vi "Test Client.vi"() -> ()   [LabVIEW 2018, in "InfluxDB Client.lvlib"]
doc: "Test program for the InfluxDB client."
uses:
  Controls/FieldSet.ctl
  Controls/TagSet.ctl
  Controls/Precision.ctl
  Classes/DataPoint/DataPoint.lvclass/DataPoint.ctl
  Classes/Results/Results.lvclass/Results.ctl
  Classes/Result/Result.lvclass/Result.ctl
  Classes/Series/Series.lvclass/Series.ctl
  InfluxDB Client.lvlib
  Classes/Client/Client.lvclass
  Classes/DataPoint/DataPoint.lvclass
  Classes/Results/Results.lvclass
  Classes/Result/Result.lvclass
  Classes/Series/Series.lvclass
panel:
  out "Tag keys":string[][][](array[string])
  out "Field keys":string[][][](array[string])
  out "Version":string
  out "Values":string[][](array[string])
  out "error out":errorcluster
  out "Measurement names":string[](array[string])
  out "Database names":string[](array[string])
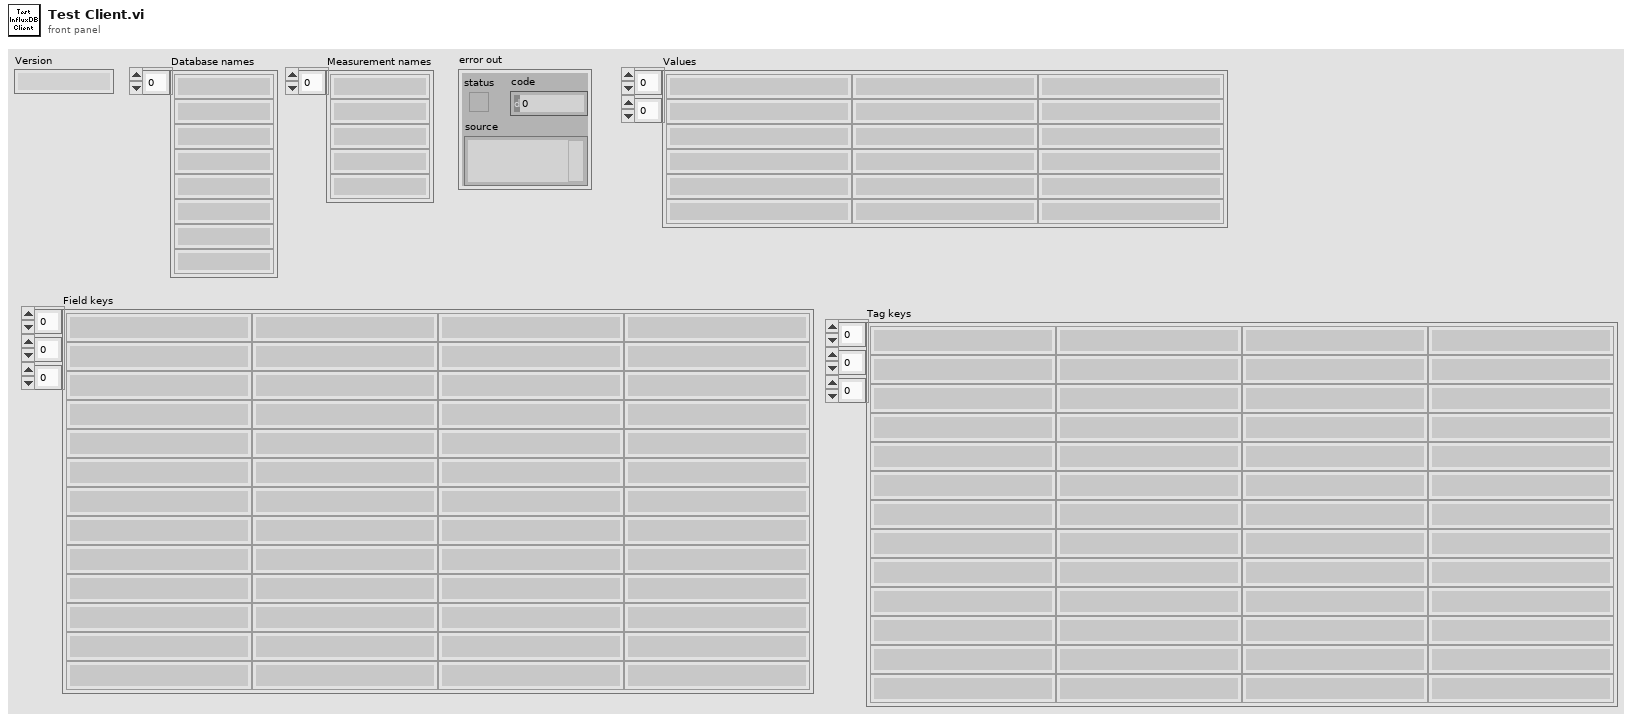
[diagram p1: front panel]
types:
  T1 = typedef "InfluxDB Client.lvlib/Precision.ctl" = enum16{"Seconds", "Milliseconds", "Nanoseconds"}
  T2 = typedef "InfluxDB Client.lvlib/TagSet.ctl" = cluster{"Key":string, "Value":string}
  T3 = typedef "InfluxDB Client.lvlib/FieldSet.ctl" = cluster{"Key":string, "Value":variant}
  T4 = typedef "Dictionary Object RefNum__ogtk.ctl" = refnum<k1>
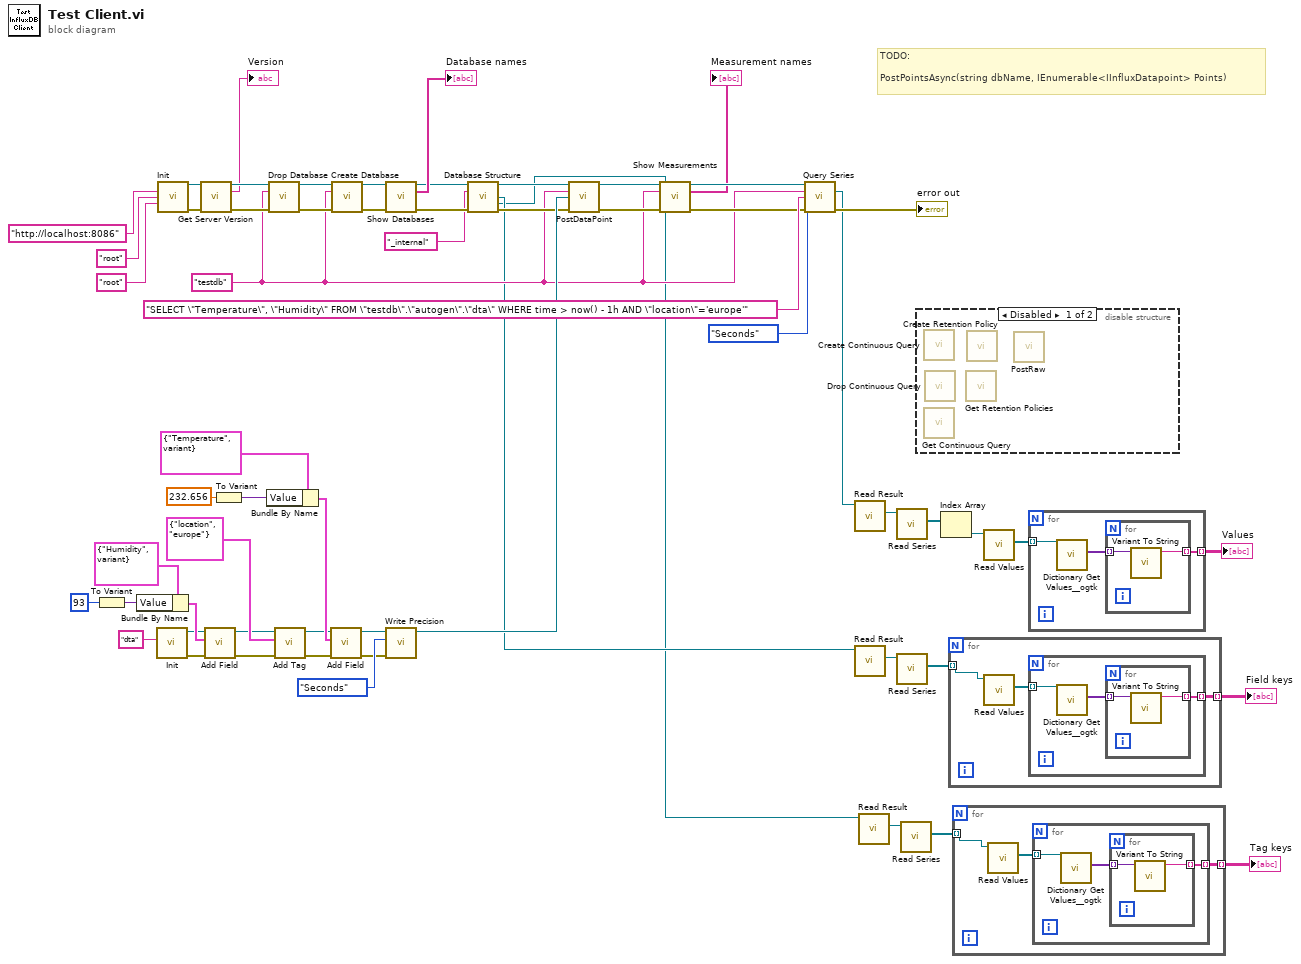
[diagram p0: block diagram]
diagram:
  w10 = "testdb" ("Database name")
  # "TODO:\n\nPostPointsAsync(string dbName, IEnumerable<IInfluxDatapoint> Points)"
  n1 = To Variant(anything=i8 93) -> (Variant=w52:variant)
  n2 = Bundle By Name(cluster=T3 {"Key"="Humidity", "Value"=variant} ("FieldSet"), "Value"=w52) -> (w51:T3)
  n3 = call "Init.vi"("Measurement"="dta") -> ("error out"=w44:errorcluster, "DataPoint out"=w45:refnum<class "DataPoint.lvclass">)  [unwired: 9 in]
  n4 = call "Init.vi"("Url"="http://localhost:8086", "Username"="root" ("Url"), "Password"="root" ("Url")) -> ("InfluxDB out"=w39:refnum<class "Client.lvclass">, "error out"=w38:errorcluster)  [unwired: 11 in]
  n5 = call "Get Server Version.vi"("InfluxDB in"=w39, "error in (no error)"=w38) -> ("InfluxDB out"=w27:refnum<class "Client.lvclass">, "Version"=→"Version":string, "error out"=w26:errorcluster)  [unwired: 11 in]
  n6 = call "Add Field.vi"("error in (no error)"=w44, "FieldSet"=w51, "DataPoint in"=w45) -> ("error out"=w42:errorcluster, "DataPoint out"=w43:refnum<class "DataPoint.lvclass">)  [unwired: 7 in]
  n7 = To Variant(anything=232.656 ("temperature")) -> (Variant=w50:variant)
  n8 = Bundle By Name(cluster=T3 {"Key"="Temperature", "Value"=variant} ("FieldSet"), "Value"=w50) -> (w46:T3)
  n9 = call "Drop Database.vi"("InfluxDB in"=w27, "Database name"=w10, "error in (no error)"=w26) -> ("InfluxDB out"=w24:refnum<class "Client.lvclass">, "error out"=w23:errorcluster)  [unwired: 11 in]
  n10 = call "Add Tag.vi"("error in (no error)"=w42, "TagSet"=T2 {"Key"="location", "Value"="europe"}, "DataPoint in"=w43) -> ("error out"=w40:errorcluster, "DataPoint out"=w41:refnum<class "DataPoint.lvclass">)  [unwired: 7 in]
  n11 = call "Add Field.vi"("error in (no error)"=w40, "FieldSet"=w46, "DataPoint in"=w41) -> ("error out"=w16:errorcluster, "DataPoint out"=w17:refnum<class "DataPoint.lvclass">)  [unwired: 7 in]
  n12 = call "Create Database.vi"("InfluxDB in"=w24, "Database name"=w10, "error in (no error)"=w23) -> ("InfluxDB out"=w57:refnum<class "Client.lvclass">, "error out"=w58:errorcluster)  [unwired: 11 in]
  n13 = call "Show Databases.vi"("InfluxDB in"=w57, "error in (no error)"=w58) -> ("InfluxDB out"=w14:refnum<class "Client.lvclass">, "Database names"=→"Database names":string[], "error out"=w12:errorcluster)  [unwired: 11 in]
  n14 = call "Write Precision.vi"("error in (no error)"=w16, "Precision"=Precision."Seconds", "DataPoint in"=w17) -> ("DataPoint out"=w29:refnum<class "DataPoint.lvclass">)  [unwired: 7 in, 1 out]
  n15 = call "Database Structure.vi"("InfluxDB in"=w14, "Database name"="_internal", "error in (no error)"=w12) -> ("InfluxDB out"=w13:refnum<class "Client.lvclass">, "Field keys"=w7:refnum<class "Results.lvclass">, "Tag keys"=w1:refnum<class "Results.lvclass">, "error out"=w11:errorcluster)  [unwired: 9 in]
  n16 = call "PostDataPoint.vi"("InfluxDB in"=w13, "Database name"=w10, "DataPoint.lvclass"=w29, "error in (no error)"=w11) -> ("InfluxDB out"=w20:refnum<class "Client.lvclass">, "error out"=w22:errorcluster)  [unwired: 10 in]
  n17 = call "Show Measurements.vi"("InfluxDB in"=w20, "Database name"=w10, "error in (no error)"=w22) -> ("InfluxDB out"=w19:refnum<class "Client.lvclass">, "Measurement names"=→"Measurement names":string[], "error out"=w21:errorcluster)  [unwired: 10 in]
  n18 = call "Query Series.vi"("InfluxDB in"=w19, "Database name"=w10, "Measurement query"="SELECT \"Temperature\", \"Humidity\" FROM \"testdb\".\"autogen\".\"dta\" WHERE time > now() - 1h AND \"location\"='europe'" ("Database name"), "Precision"=Precision."Seconds", "error in (no error)"=w21) -> ("Results Out"=w15:refnum<class "Results.lvclass">, "error out"=→"error out":errorcluster)  [unwired: 8 in, 1 out]
  n19 = call "Read Result.vi"("Results in"=w15) -> ("Result.lvclass"=w35:refnum<class "Result.lvclass">)  [unwired: 9 in, 1 out]
  n20 = call "Read Result.vi"("Results in"=w7) -> ("Result.lvclass"=w9:refnum<class "Result.lvclass">)  [unwired: 9 in, 1 out]
  n21 = call "Read Result.vi"("Results in"=w1) -> ("Result.lvclass"=w4:refnum<class "Result.lvclass">)  [unwired: 9 in, 1 out]
  n22 = call "Read Series.vi"("Result in"=w35) -> ("Series"=w34:refnum<class "Series.lvclass">[])  [unwired: 9 in, 1 out]
  n23 = call "Read Series.vi"("Result in"=w9) -> ("Series"=w5:refnum<class "Series.lvclass">[])  [unwired: 9 in, 1 out]
  n24 = call "Read Series.vi"("Result in"=w4) -> ("Series"=w2:refnum<class "Series.lvclass">[])  [unwired: 9 in, 1 out]
  n25 = disable-structure shown="Disabled" {
    frame Disabled {
      n26 = call "Create Continuous Query.vi"() -> ()  [unwired: 14 in, 2 out]
      n27 = call "Get Continuous Query.vi"() -> ()  [unwired: 13 in, 3 out]
      n28 = call "Drop Continuous Query.vi"() -> ()  [unwired: 14 in, 2 out]
      n29 = call "Get Retention Policies.vi"() -> ()  [unwired: 13 in, 3 out]
      n30 = call "Create Retention Policy.vi"() -> ()  [unwired: 14 in, 2 out]
      n31 = call "PostRaw.vi"() -> ()  [unwired: 14 in, 2 out]
    }
    frame Enabled {
    }
  }
  n32 = Index Array(array=w34) -> (element=w33:refnum<class "Series.lvclass">)  [unwired: 1 in]
  n33 = for {
    tunnel: [w63] -> w8 mode=indexing
    tunnel: w5 -> [w62] mode=indexing
    n34 = call "Read Values.vi"("Series in"=w62) -> ("Values"=w64:T4[])  [unwired: 9 in, 1 out]
    n35 = for {
      tunnel: w64 -> [w67] mode=indexing
      tunnel: [w65] -> w63 mode=indexing
      n36 = call <userlib>:"Dictionary Get Values__ogtk.vi"("dictionary"=w67) -> ("values"=w66:variant[])  [unwired: 8 in, 2 out]
      n37 = for {
        tunnel: w66 -> [w69] mode=indexing
        tunnel: [w68] -> w65 mode=indexing
        n38 = call "Variant To String.vi"("Variant"=w69) -> ("String"=w68:string)  [unwired: 9 in, 1 out]
      }
    }
  }
  "Field keys" <- w8
  n39 = for {
    tunnel: [w71] -> w3 mode=indexing
    tunnel: w2 -> [w70] mode=indexing
    n40 = call "Read Values.vi"("Series in"=w70) -> ("Values"=w72:T4[])  [unwired: 9 in, 1 out]
    n41 = for {
      tunnel: w72 -> [w75] mode=indexing
      tunnel: [w73] -> w71 mode=indexing
      n42 = call <userlib>:"Dictionary Get Values__ogtk.vi"("dictionary"=w75) -> ("values"=w74:variant[])  [unwired: 8 in, 2 out]
      n43 = for {
        tunnel: w74 -> [w77] mode=indexing
        tunnel: [w76] -> w73 mode=indexing
        n44 = call "Variant To String.vi"("Variant"=w77) -> ("String"=w76:string)  [unwired: 9 in, 1 out]
      }
    }
  }
  "Tag keys" <- w3
  n45 = call "Read Values.vi"("Series in"=w33) -> ("Values"=w32:T4[])  [unwired: 9 in, 1 out]
  n46 = for {
    tunnel: w32 -> [w80] mode=indexing
    tunnel: [w78] -> w31 mode=indexing
    n47 = call <userlib>:"Dictionary Get Values__ogtk.vi"("dictionary"=w80) -> ("values"=w79:variant[])  [unwired: 8 in, 2 out]
    n48 = for {
      tunnel: w79 -> [w82] mode=indexing
      tunnel: [w81] -> w78 mode=indexing
      n49 = call "Variant To String.vi"("Variant"=w82) -> ("String"=w81:string)  [unwired: 9 in, 1 out]
    }
  }
  "Values" <- w31
